vi "Initialize (Simulator).vi"(8 "error in (no error)":errorcluster, 11 "Device ID":T1) -> (0 "error out":errorcluster, 3 "DC Motor Controller out":refnum<class "DC Motor Controller.lvclass">)   [LabVIEW 2019, in "DC Motor Controller Simulator.lvclass"]
doc: "Establishes communication with the sensor. Therefore, call this VI before calling other sensor driver VIs for this sensor. Generally, you need to call the Initialize VI only once at the beginning of an application.\n\n<B>Note:</B>\nYou must call the Start Simulator Service VI on the <B>Robotics>>Simulator</B> palette before calling this VI."
uses:
  DC Motor Controller Simulator.lvclass
  <vilib>/robotics/Simulator/NI_Robotics_Simulator.lvlib
  DC Motor Controller.lvclass
  <vilib>/robotics/Simulator/Engine/ctl/DeviceID.ctl
panel:
  # "(c) 2011 National Instruments.  ALL RIGHTS RESERVED."
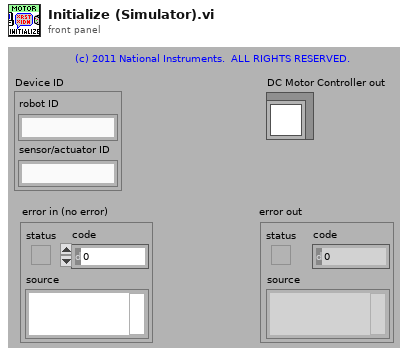
[diagram p1: front panel]
types:
  T1 = typedef "NI_Robotics_Simulator.lvlib/DeviceID.ctl" = cluster{"robot ID":string, "sensor/actuator ID":string}
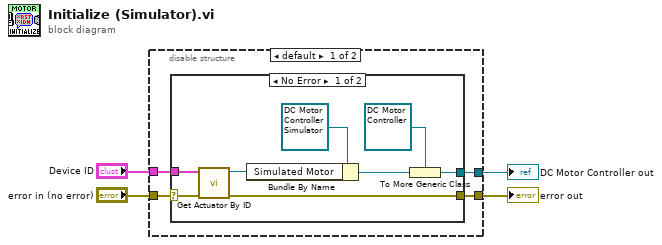
[diagram p0: block diagram]
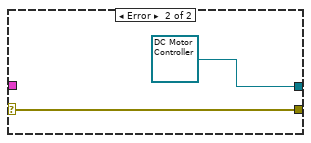
[diagram p2: hidden frame]
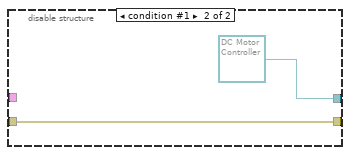
[diagram p3: hidden frame]
diagram:
  n1 = disable-structure shown="default" {
    disable-tunnel: "Device ID" -> [w8 _]
    disable-tunnel: "error in (no error)" -> [w7 w20]
    disable-tunnel: [w6 refnum<class "DC Motor Controller.lvclass"> refnum ("target class")] -> w2
    disable-tunnel: [w5 w20] -> w1
    frame condition #0 (active) {
      n2 = case shown="No Error" w7 {
        selector: w7 -> [w14 w18]
        tunnel: [w13 w18] -> w5
        tunnel: [w9 refnum<class "DC Motor Controller.lvclass"> refnum ("target class")] -> w6
        tunnel: w8 -> [w15 _]
        frame No Error {
          n3 = call <vilib>:"Get Actuator By ID.vi"("error in (no error)"=w14, "device ID"=w15) -> ("error out"=w13:errorcluster, "actuator class"=w12:refnum<class "ODESimulator_Motor.lvclass">)  [unwired: 8 in]
          n4 = Bundle By Name(cluster=refnum<class "DC Motor Controller Simulator.lvclass"> refnum ("Starter Kit Motor Controller Simulator.lvclass"), "Simulated Motor"=w12) -> (w11:refnum<class "DC Motor Controller Simulator.lvclass">)
          n5 = To More Generic Class(target class=refnum<class "DC Motor Controller.lvclass"> refnum, reference=w11) -> (generic class reference=w9:refnum<class "DC Motor Controller.lvclass">)
        }
        frame Error {
        }
      }
    }
    frame condition #1 {
    }
  }
  "error out" <- w1
  "DC Motor Controller out" <- w2
